vi "Get Database Errors.vi"(0 "My Errors":errorcluster, 1 "ADO Open Errors":errorcluster, 6 "Connection In":refnum<k7>) -> (2 "error out":errorcluster, 8 "Connection Out":refnum<k7>)   [LabVIEW 2020, in "hse-db-ado.lvlib" / "ADO-DB-Driver.lvlib"]
doc: "Get database errors\n\n____\nHAMPEL SOFTWARE ENGINEERING v1.4.0 (2023-12-19 09:52)"
uses:
  ADO-DB-Driver.lvlib
panel:
  # "This VI tries to get more information on an event based on the ADO connection.error collection. There is no guarantee that it will get anything more, but it at least tries..."
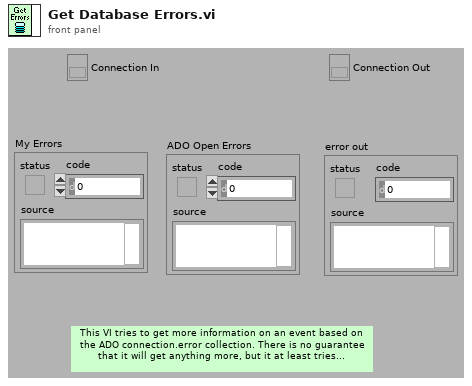
[diagram p1: front panel]
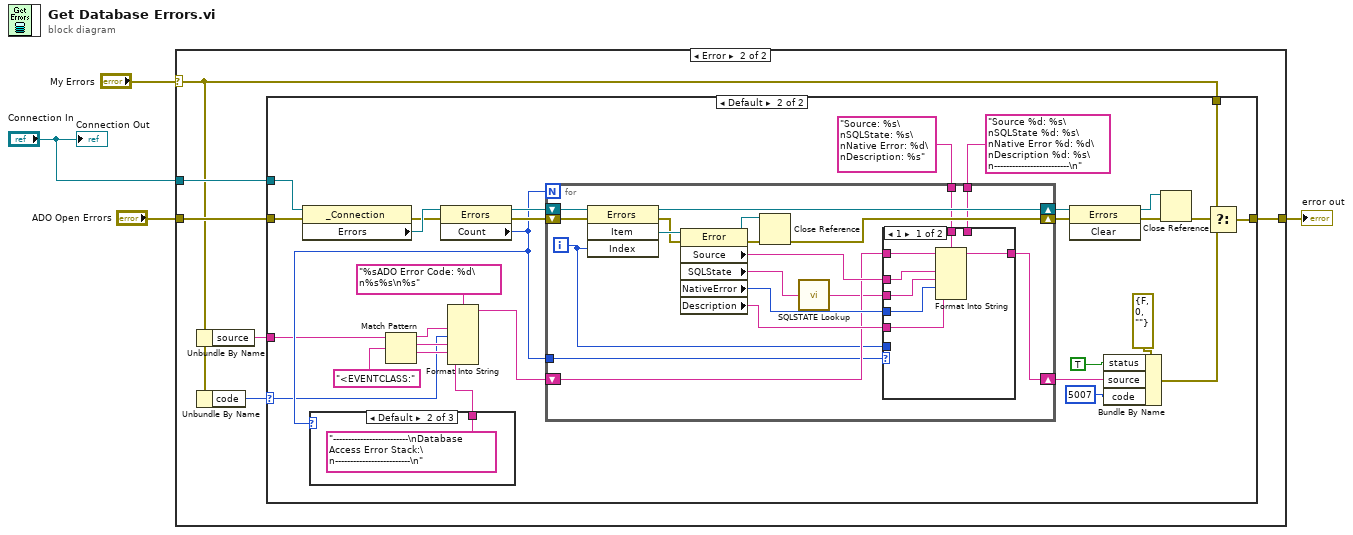
[diagram p0: block diagram]
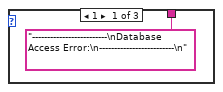
[diagram p4: hidden frame]
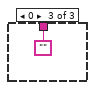
[diagram p5: hidden frame]
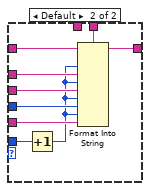
[diagram p6: hidden frame]
diagram:
  n1 = case shown="Error" "My Errors" {
    selector: "My Errors" -> [_ w6]
    tunnel: "Connection In" -> [_ w11]
    tunnel: "ADO Open Errors" -> [w5 w10]
    tunnel: [w5 w9] -> w4
    frame No Error {
    }
    frame Error {
      n2 = Unbundle By Name(w6) -> ("source"=w7:string)
      n3 = Unbundle By Name(w6) -> ("code"=w8:i32)
      n4 = case shown="Default" w8 {
        selector: w8 -> [_ w16]
        tunnel: w11 -> [_ w42]
        tunnel: w10 -> [_ w37]
        tunnel: [w12 w36] -> w9
        tunnel: w6 -> [w12 w22]
        tunnel: w7 -> [_ w15]
        frame 5000..9999 {
        }
        frame Default {
          n5 = property class="_Connection"(reference=w42, error in=w37) -> (error out=w38:errorcluster, "Errors"=w41:refnum<k7>)  [unwired: 1 out]
          n6 = Match Pattern(string=w15, regular expression="<EVENTCLASS:") -> (before substring=w19:string, match substring=w20:string, after substring=w21:string)  [unwired: 1 in, 1 out]
          n7 = property class="Errors"(reference=w41, error in=w38) -> (reference out=w40:refnum<k7>, error out=w39:errorcluster, "Count"=w31:i32)
          n8 = case shown="Default" w31 {
            tunnel: ["-------------------------\nDatabase Access Error:\n-------------------------\n" "-------------------------\nDatabase Access Error Stack:\n-------------------------\n" ""] -> w13
            frame 1 {
            }
            frame Default {
            }
            frame 0 {
            }
          }
          n9 = Format Into String(format string="%sADO Error Code: %d\n%s%s\n%s", w19, w16, w20, w21, w13) -> (resulting string=w17:string)  [unwired: 2 in, 1 out]
          n10 = for {
            N: w31 -> [_]
            shift-right: [w58] -> w25
            shift-left: w39 -> [w63]
            shift-right: [w57] -> w26
            shift-left: w40 -> [w64]
            shift-right: [w49] -> w34
            shift-left: w17 -> [w53]
            tunnel: w31 -> [w52]
            tunnel: "Source: %s\nSQLState: %s\nNative Error: %d\nDescription: %s" -> [w50]
            tunnel: "Source %d: %s\nSQLState %d: %s\nNative Error %d: %d\nDescription %d: %s\n-------------------------\n" -> [w48]
            i -> [w51]
            n11 = invoke class="Errors" method="Item"(reference=w64, error in=w63, "Index"=w51) -> (reference out=w57:refnum<k7>, error out=w61:errorcluster, "Item"=w62:refnum<k7>)  [unwired: 1 in, 1 out]
            n12 = property class="Error"(reference=w62, error in=w61) -> (reference out=w59:refnum<k7>, error out=w60:errorcluster, "Source"=w54:string, "SQLState"=w47:string, "NativeError"=w55:i32, "Description"=w56:string)
            n13 = Close Reference(reference=w59, error in (no error)=w60) -> (error out=w58:errorcluster)
            n14 = call "SQLSTATE Lookup.vi"("SQLSTATE Value"=w47) -> ("SQLSTATE Description"=w46:string)  [unwired: 4 in]
            n15 = case shown="1" w52 {
              tunnel: w56 -> [w71 w77]
              tunnel: w55 -> [w66 w76]
              tunnel: w54 -> [w65 w73]
              tunnel: w53 -> [w69 w80]
              tunnel: w51 -> [_ w74]
              tunnel: w50 -> [w70 _]
              tunnel: [w68 w79] -> w49
              tunnel: w48 -> [_ w78]
              tunnel: w46 -> [w67 w75]
              frame 1 {
                n16 = Format Into String(format string=w70, initial string=w69, w65, w67, w66, w71) -> (resulting string=w68:string)  [unwired: 1 in, 1 out]
              }
              frame Default {
                n17 = Increment(x=w74) -> (x+1=w72:i32)
                n18 = Format Into String(format string=w78, initial string=w80, w72, w73, w72, w75, w72, w76, w72, w77) -> (resulting string=w79:string)  [unwired: 1 in, 1 out]
              }
            }
          }
          n19 = invoke class="Errors" method="Clear"(reference=w26, error in=w25) -> (reference out=w24:refnum<k7>, error out=w23:errorcluster)  [unwired: 1 in, 1 out]
          n20 = Bundle By Name(cluster=errorcluster {"status"=FALSE, "code"=0, "source"=""} ("error out"), "status"=TRUE, "source"=w34, "code"=5007) -> (w35:errorcluster)
          n21 = Close Reference(reference=w24, error in (no error)=w23) -> (error out=w27:errorcluster)
          n22 = Select(t=w22, s=w27, f=w35) -> (s? t:f=w36:errorcluster)
        }
      }
    }
  }
  "error out" <- w4
  "Connection Out" <- "Connection In"
